vi "Query FM Properties.vi"(0 "VISA resource name":refnum<visa-resource-name>, 5 "Channel (0: Channel 1)":T1 items=["Channel 1", "Channel 2"], 11 "error in (no error)":errorcluster) -> (4 "VISA resource name out":refnum<visa-resource-name>, 6 "FM Source":u16(ring) items=["Internal", "External"], 8 "Modulation Waveform":u16(ring) items=["Sine", "Square", "Triangle", "Ramp", "Down Ramp", "Noise", "User 1", "User 2", "User 3", "User 4", "EMEMory", "EFILe"], 10 "Modulation Frequency":dbl[unit]=100.0, 14 "Peak Deviation":dbl[unit]=100.0, 15 "error out":errorcluster)   [LabVIEW 2023, in "Tektronix AFG 3000 Series.lvlib"]
uses:
  Tektronix AFG 3000 Series.lvlib
  controls.llb/Channel.ctl
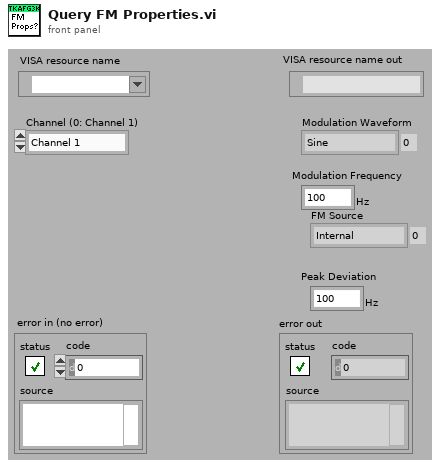
[diagram p1: front panel]
types:
  T1 = typedef "Channel.ctl" = u16
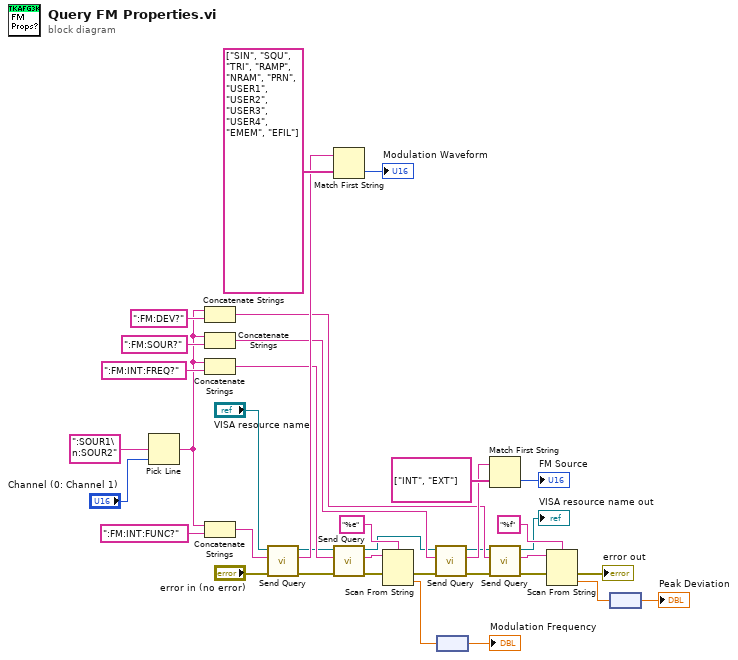
[diagram p0: block diagram]
diagram:
  n1 = Pick Line(multi-line string=":SOUR1\n:SOUR2" ("string (\"\")"), line index="Channel (0: Channel 1)") -> (output string=w16:string)  [unwired: 1 out]
  n2 = Concatenate Strings(w16, ":FM:DEV?" ("string")) -> (w17:string)
  n3 = Concatenate Strings(w16, ":FM:SOUR?" ("string")) -> (w24:string)
  n4 = Concatenate Strings(w16, ":FM:INT:FREQ?" ("string")) -> (w31:string)
  n5 = Concatenate Strings(w16, ":FM:INT:FUNC?" ("string")) -> (w34:string)
  n6 = call "Send Query.vi"("error in (no error)"="error in (no error)", "write buffer"=w34, "VISA resource name"="VISA resource name") -> ("error out"=w27:errorcluster, "read buffer"=w33:string, "VISA resource name out"=w26:refnum<visa-resource-name>)  [unwired: 1 in, 5 out]
  n7 = Match First String(2:string[] ["SIN", "SQU", "TRI", "RAMP", "NRAM", "PRN", "USER1", "USER2", "USER3", "USER4", "EMEM", "EFIL"], 3:w33) -> (0:→"Modulation Waveform":i32)  [unwired: 1 out]
  n8 = call "Send Query.vi"("error in (no error)"=w27, "write buffer"=w31, "VISA resource name"=w26) -> ("error out"=w21:errorcluster, "read buffer"=w29:string, "VISA resource name out"=w12:refnum<visa-resource-name>)  [unwired: 1 in, 5 out]
  n9 = Scan From String(format string="%e", input string=w29, error in=w21) -> (error out=w20:errorcluster, output 1=w28:dbl)  [unwired: 1 in, 3 out]
  n10 = call "Send Query.vi"("error in (no error)"=w20, "write buffer"=w24, "VISA resource name"=w12) -> ("error out"=w19:errorcluster, "read buffer"=w22:string, "VISA resource name out"=w11:refnum<visa-resource-name>)  [unwired: 1 in, 5 out]
  n11 = node(w28) -> (→"Modulation Frequency":dbl[unit])
  n12 = Match First String(2:string[] ["INT", "EXT"], 3:w22) -> (0:→"FM Source":i32)  [unwired: 1 out]
  n13 = call "Send Query.vi"("error in (no error)"=w19, "write buffer"=w17, "VISA resource name"=w11) -> ("error out"=w14:errorcluster, "read buffer"=w13:string, "VISA resource name out"=→"VISA resource name out":refnum<visa-resource-name>)  [unwired: 1 in, 5 out]
  n14 = Scan From String(format string="%f", input string=w13, error in=w14) -> (error out=→"error out":errorcluster, output 1=w6:dbl)  [unwired: 2 in, 2 out]
  n15 = node(w6) -> (→"Peak Deviation":dbl[unit])
